vi "Test StateMachine API.vi"() -> ()   [LabVIEW 2020]
doc: "StateMachine API Tester.\n\n<b>Note:</b> This VI was modified by the <b>Validate DQMH Module</b> tool to add the 'Show Main VI Diagram on Init' functionality included in DQMH 6.1.\n\n<b>Note:</b> This VI was modified by the <b>Validate DQMH Module</b> tool to upgrade its Error Reported event frame to use an improved mechanism for displaying error information.\n\n____\nHAMPEL SOFTWARE ENGINEERING v2.6.0 (2023-12-19 10:54)"
uses:
  Libraries/hse-libraries/Source/hse-dqmh/Controls/Module Display Scenarios.ctl
  HSE-SM/SM_Transitions.ctl
  <vilib>/Utility/error.llb/DialogType.ctl
  <vilib>/Hampel Software Engineering/HSE Logger/LogRecord/LogRecord.lvclass/LogRecord.ctl
  StateMachine.lvlib
  Libraries/hse-libraries/Source/hse-dqmh/hse-dqmh.lvlib
  <vilib>/Hampel Software Engineering/HSE Logger/LogRecord/LogRecord.lvclass
  <vilib>/Hampel Software Engineering/HSE Logger/hse-logger.lvlib
  HSE-SM/HSE-State-Machine.lvlib
panel:
  in  "Show Main VI Diagram on Init (F)":bool
  in  "DEMO Transition to inject":T1
  in  "DEMO Inject Transition":bool
  in  "Scenario":T2
  in  "Request UI Display":bool
  in  "Prepare":bool
  in  "Configure":bool
  in  "Show Block Diagram":bool
  in  "Stop Module":bool
  in  "Start Module":bool
  in  "Hide Module Panel":bool
  in  "Show Module Panel":bool
  out "Status":string
  out "Module Running?":bool
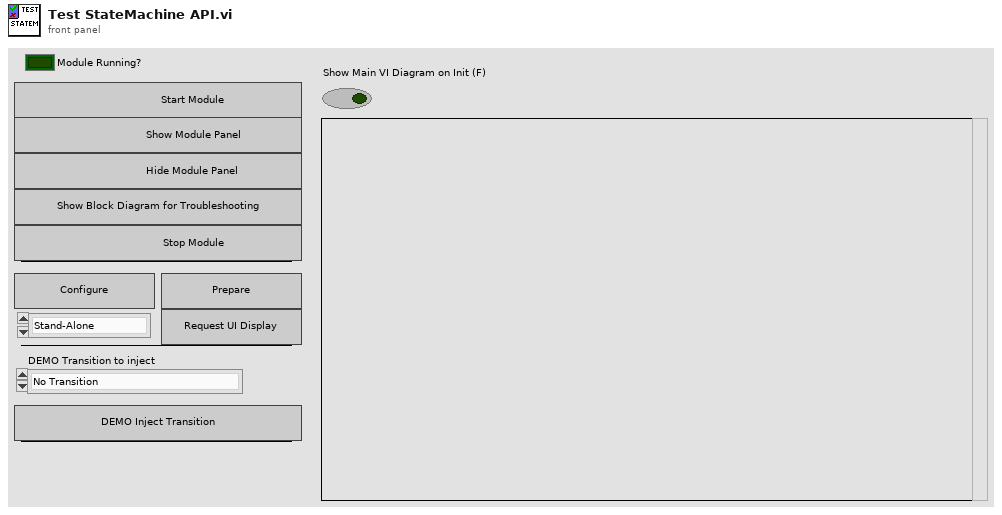
[diagram p1: front panel]
types:
  T1 = typedef "StateMachine.lvlib/HSE-State-Machine.lvlib/SM_Transitions.ctl" = enum16{"No Transition", "Exception", "Reset", "Initialization finished", "Process started", "Trigger detected", "Exit"}
  T2 = typedef "hse-dqmh.lvlib/Module Display Scenarios.ctl" = enum16{"Stand-Alone", "Managed"}
  T3 = typedef "StateMachine.lvlib/Broadcast Events--cluster.ctl" = cluster{"Module Did Init":refnum<user-event>, "Status Updated":refnum<user-event>, "Error Reported":refnum<user-event>, "Module Did Stop":refnum<user-event>, "Update Module Execution Status":refnum<user-event>, "System Message":refnum<user-event>, "DEMO Updated UI State":refnum<user-event>}
  T4 = typedef "DialogType.ctl" = u16
  T5 = typedef "hse-dqmh.lvlib/System Message Source.ctl" = enum16{"module", "application", "network"}
  T6 = typedef "hse-logger.lvlib/LogLevel.ctl" = enum16{"DEBUG", "INFO", "WARNING", "ERROR", "CRITICAL"}
  T7 = typedef "StateMachine.lvlib/HSE-State-Machine.lvlib/SM_States.ctl" = enum16{"No State - Error", "Error - Waiting For Action", "Initialising", "Standing by (idle)", "Waiting for External Trigger", "Polling for Signal Change", "Exiting"}
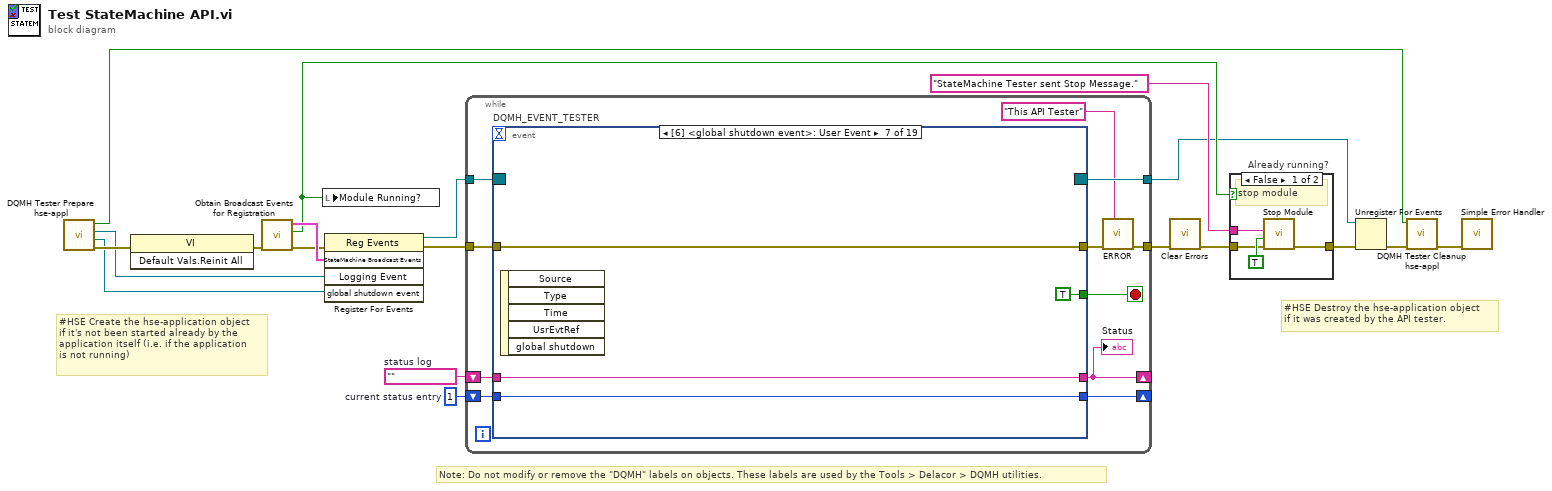
[diagram p0: block diagram]
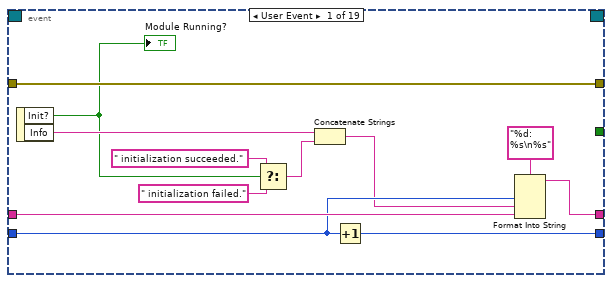
[diagram p3: hidden frame]
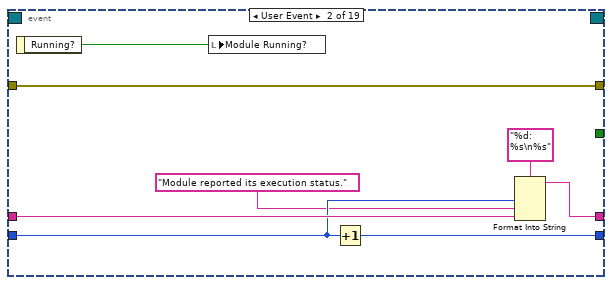
[diagram p4: hidden frame]
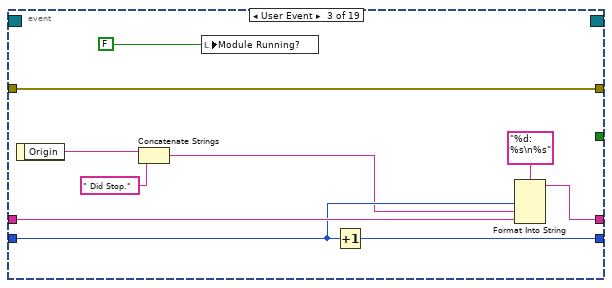
[diagram p5: hidden frame]
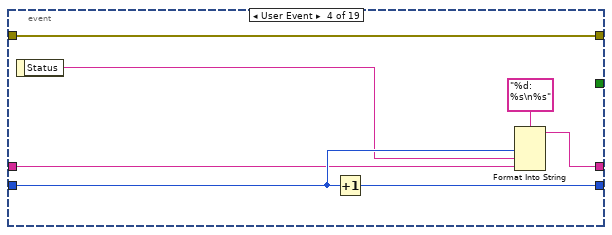
[diagram p6: hidden frame]
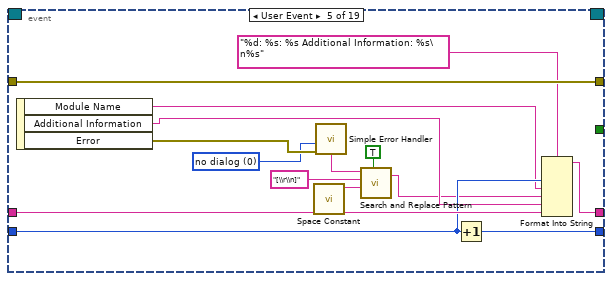
[diagram p7: hidden frame]
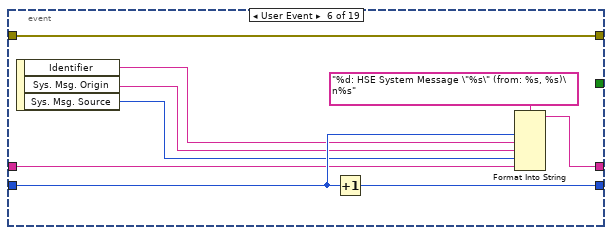
[diagram p8: hidden frame]
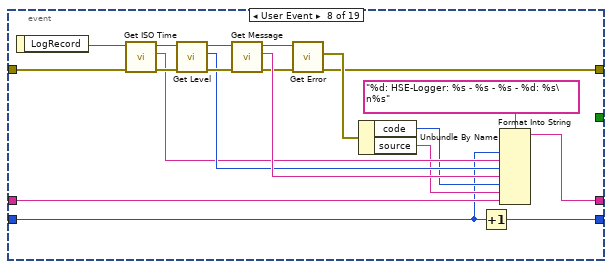
[diagram p9: hidden frame]
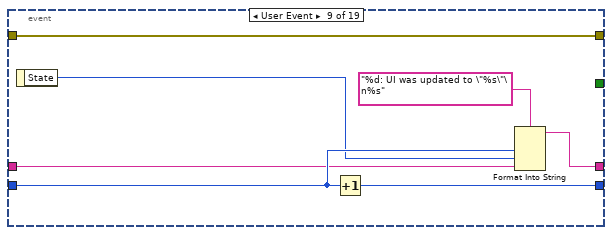
[diagram p10: hidden frame]
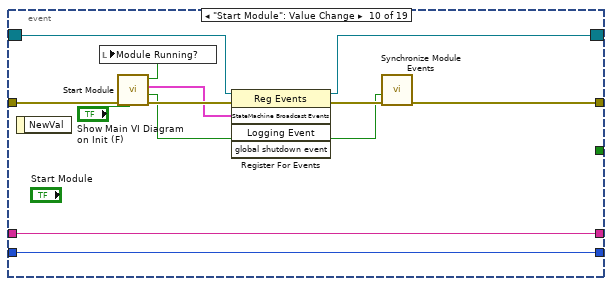
[diagram p11: hidden frame]
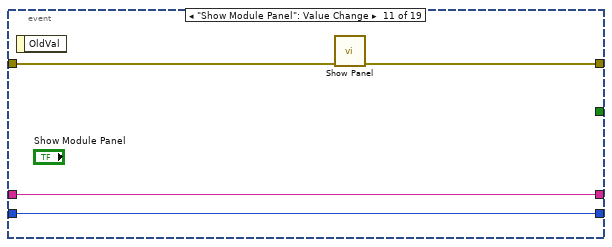
[diagram p12: hidden frame]
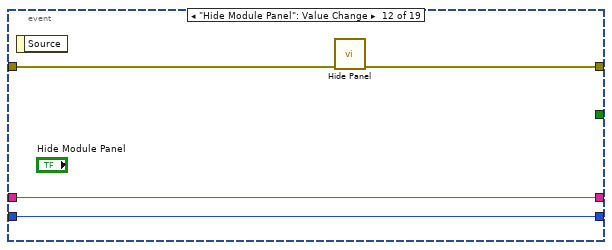
[diagram p13: hidden frame]
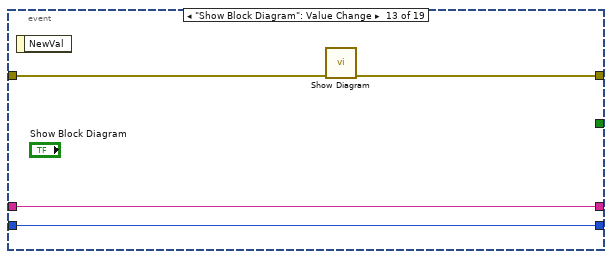
[diagram p14: hidden frame]
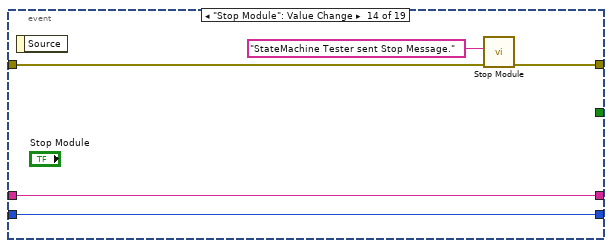
[diagram p15: hidden frame]
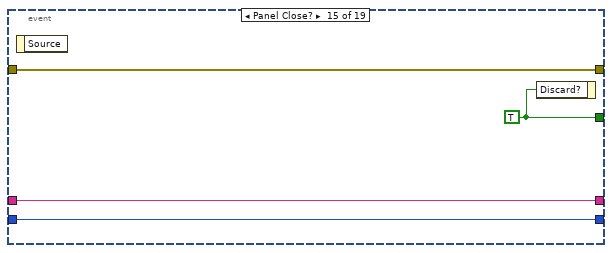
[diagram p16: hidden frame]
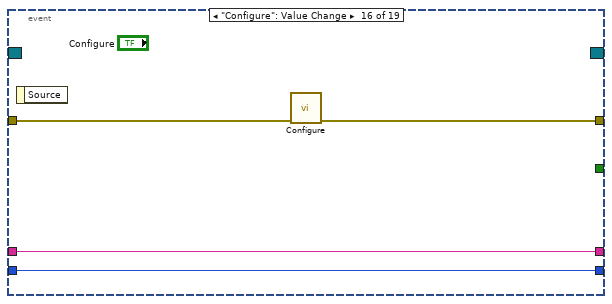
[diagram p17: hidden frame]
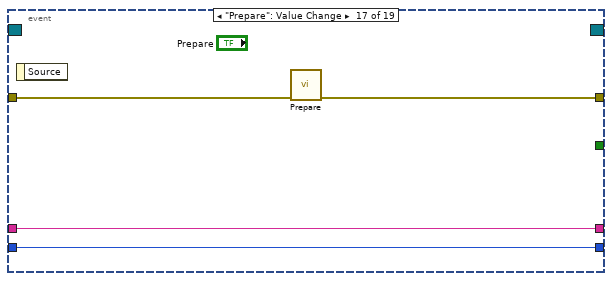
[diagram p18: hidden frame]
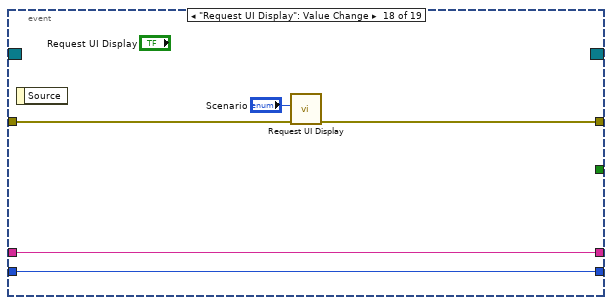
[diagram p19: hidden frame]
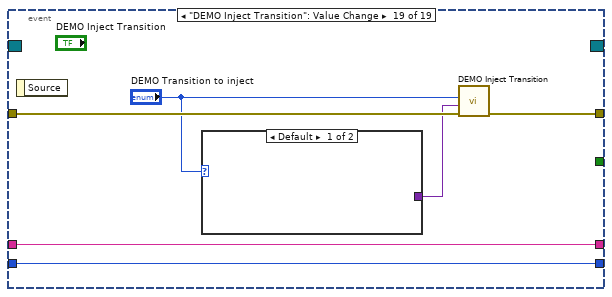
[diagram p20: hidden frame]
diagram:
  w15 = 1  # current status entry
  w16 = ""  # status log
  # "#HSE Destroy the hse-application object\nif it was created by the API tester."
  # "#HSE Create the hse-application object\nif it's not been started already by the \napplication itself (i.e. if the application\nis not running)"
  # "Note: Do not modify or remove the \"DQMH\" labels on objects. These labels are used by the Tools > Delacor > DQMH utilities."
  n1 = call "DQMH Tester Prepare hse-appl.vi"() -> ("error out"=w6:errorcluster, "global shutdown event"=w1:refnum<user-event>, "Logging Event"=w5:refnum<user-event>, "Started?"=w4:bool)  [unwired: 8 in]
  n2 = invoke class="VI" method="Default Vals.Reinit All"(error in=w6) -> (error out=w9:errorcluster)  [unwired: 2 in, 2 out]
  n3 = call "Obtain Broadcast Events for Registration.vi"("error in (no error)"=w9) -> ("error out"=w8:errorcluster, "Already running?"=w7:bool, "StateMachine Broadcast Events"=w13:T3)  [unwired: 8 in]
  n4 = local write "Module Running?"(w7) -> ()
  n5 = register-events(error in=w8, w13, w5, w1) -> (reference out=w12:refnum<event-registration>, error out=w14:errorcluster)  [unwired: 1 in]
  n6 = while {
    tunnel: w12 -> [w30]
    tunnel: [w21] -> w10
    shift-right: [w26] -> _
    shift-left: w16 -> [w28]
    shift-right: [w27] -> _
    shift-left: w15 -> [w29]
    tunnel: w14 -> [w25]
    tunnel: [w24] -> w2
    stop <- w23 stop-if-true
    n7 = event "DQMH_EVENT_TESTER" shown="[6] <global shutdown event>: User Event" {
      selector: w30 -> [_ _ _ _ _ _ _ _ _ w127 _ _ _ _ _ _ _ _ _]
      dyn-events: [_ _ _ _ _ _ _ _ _ w126 _ _ _ _ _ _ _ _ _] -> w24
      timeout: _ -> [_ _ _ _ _ _ _ _ _ _ _ _ _ _ _ _ _ _ _]
      tunnel: [_ _ _ _ _ _ TRUE ("Discard?") _ _ _ _ _ _ _ w154 _ _ _ _] -> w23
      tunnel: [w42 w44 w51 w61 w82 w86 w95 w96 w121 w125 w137 w141 w142 w148 w151 w155 w159 w164 w170] -> w22
      tunnel: w29 -> [w39 w48 w58 w64 w79 w88 w93 w99 w120 w130 w135 w139 w143 w149 w152 w156 w160 w165 w171]
      tunnel: w28 -> [w40 w49 w59 w63 w81 w85 w94 w100 w118 w131 w136 w140 w144 w150 w153 w157 w161 w166 w172]
      tunnel: [w37 w46 w56 w65 w80 w89 w94 w97 w117 w131 w136 w140 w144 w150 w153 w157 w161 w166 w172] -> w26
      tunnel: [w38 w47 w57 w67 w78 w91 w93 w98 w120 w130 w135 w139 w143 w149 w152 w156 w160 w165 w171] -> w27
      tunnel: w25 -> [w42 w44 w51 w61 w82 w86 w95 w102 w121 w124 w134 w138 w145 w146 w151 w158 w162 w167 w173]
      event User Event {
        n8 = event-data() -> ("Init?"=w34:bool, "Info"=w36:string)  [unwired: 1 in]
        "Module Running?" <- w34
        n9 = Select(t=" initialization succeeded.", s=w34, f=" initialization failed.") -> (s? t:f=w31:string)
        n10 = Concatenate Strings(w36, w31) -> (w35:string)
        n11 = Increment(x=w39) -> (x+1=w38:i32)
        n12 = Format Into String(format string="%d: %s\n%s", w39, w35, w40) -> (resulting string=w37:string)  [unwired: 2 in, 1 out]
      }
      event User Event {
        n13 = event-data() -> ("Running?"=w43:bool)  [unwired: 1 in]
        n14 = local write "Module Running?"(w43) -> ()
        n15 = Increment(x=w48) -> (x+1=w47:i32)
        n16 = Format Into String(format string="%d: %s\n%s", w48, "Module reported its execution status.", w49) -> (resulting string=w46:string)  [unwired: 2 in, 1 out]
      }
      event User Event {
        n17 = event-data() -> ("Origin"=w55:string)  [unwired: 1 in]
        n18 = Concatenate Strings(w55, " Did Stop.") -> (w54:string)
        n19 = local write "Module Running?"(FALSE ("Module Did Init?")) -> ()
        n20 = Increment(x=w58) -> (x+1=w57:i32)
        n21 = Format Into String(format string="%d: %s\n%s", w58, w54, w59) -> (resulting string=w56:string)  [unwired: 2 in, 1 out]
      }
      event User Event {
        n22 = event-data() -> ("Status"=w62:string)  [unwired: 1 in]
        n23 = Increment(x=w64) -> (x+1=w67:i32)
        n24 = Format Into String(format string="%d: %s\n%s", w64, w62, w63) -> (resulting string=w65:string)  [unwired: 2 in, 1 out]
      }
      event User Event {
        w74 = T4 0 items=["no dialog", "OK message", "continue or stop message", "OK message + warnings", "continue/stop + warnings"] ("type of dialog (OK msg:1)")
        n25 = event-data() -> ("Module Name"=w75:string, "Additional Information"=w76:string, "Error"=w77:errorcluster)  [unwired: 1 in]
        n26 = call <vilib>:"Space Constant.vi"() -> ("String"=w70:string)
        n27 = call <vilib>:"Simple Error Handler.vi"("type of dialog (OK msg:1)"=w74, "error in (no error)"=w77) -> ("message"=w73:string)  [unwired: 3 in, 4 out]
        n28 = call <vilib>:"Search and Replace Pattern.vi"("string"=w73, "regular expression (\"\")"="[\\r\\n]" ("regular expression (\"\")"), "replace string (\"\")"=w70, "replace all? (F)"=TRUE ("replace all CR/LF with spaces")) -> ("result string"=w72:string)  [unwired: 1 in, 1 out]
        n29 = Increment(x=w79) -> (x+1=w78:i32)
        n30 = Format Into String(format string="%d: %s: %s Additional Information: %s\n%s", w79, w75, w72, w76, w81) -> (resulting string=w80:string)  [unwired: 2 in, 1 out]
      }
      event User Event {
        n31 = event-data() -> ("Identifier"=w87:string, "Sys. Msg. Origin"=w83:string, "Sys. Msg. Source"=w84:T5)  [unwired: 1 in]
        n32 = Increment(x=w88) -> (x+1=w91:i32)
        n33 = Format Into String(format string="%d: HSE System Message \"%s\" (from: %s, %s)\n%s", w88, w87, w83, w84, w85) -> (resulting string=w89:string)  [unwired: 2 in, 1 out]
      }
      event User Event {
        n34 = event-data() -> ()  [unwired: 1 in, 5 out]
      }
      event User Event {
        n35 = event-data() -> ("LogRecord"=w101:refnum<class "LogRecord.lvclass">)  [unwired: 1 in]
        n36 = call <vilib>:"Get ISO Time.vi"("error in"=w102, "LogRecord in"=w101) -> ("error out"=w107:errorcluster, "ISO Time"=w106:string, "LogRecord out"=w109:refnum<class "LogRecord.lvclass">)  [unwired: 7 in]
        n37 = call <vilib>:"Get Level.vi"("error in"=w107, "LogRecord in"=w109) -> ("error out"=w110:errorcluster, "Level"=w108:T6, "LogRecord out"=w111:refnum<class "LogRecord.lvclass">)  [unwired: 7 in]
        n38 = call <vilib>:"Get Message.vi"("error in"=w110, "LogRecord in"=w111) -> ("error out"=w112:errorcluster, "Message"=w115:string, "LogRecord out"=w113:refnum<class "LogRecord.lvclass">)  [unwired: 7 in]
        n39 = call <vilib>:"Get Error.vi"("error in"=w112, "LogRecord in"=w113) -> ("error out"=w96:errorcluster, "Error"=w114:errorcluster)  [unwired: 7 in, 1 out]
        n40 = Unbundle By Name(w114) -> ("code"=w104:i32, "source"=w105:string)
        n41 = Increment(x=w99) -> (x+1=w98:i32)
        n42 = Format Into String(format string="%d: HSE-Logger: %s - %s - %s - %d: %s\n%s", w99, w106, w108, w115, w104, w105, w100) -> (resulting string=w97:string)  [unwired: 2 in, 1 out]
      }
      event User Event {
        n43 = event-data() -> ("State"=w119:T7)  [unwired: 1 in]
        n44 = Increment(x=w120) -> ()  [unwired: 1 out]
        n45 = Format Into String(format string="%d: UI was updated to \"%s\"\n%s", w120, w119, w118) -> (resulting string=w117:string)  [unwired: 2 in, 1 out]
      }
      event "Start Module": Value Change {
        n46 = event-data() -> ()  [unwired: 1 in, 1 out]
        n47 = call "Start Module.vi"("Show Main VI Diagram on Init (F)"="Show Main VI Diagram on Init (F)", "error in (no error)"=w124) -> ("error out"=w132:errorcluster, "Wait for Event Sync?"=w129:bool, "StateMachine Broadcast Events"=w128:T3, "Module Was Already Running?"=w123:bool)  [unwired: 6 in]
        n48 = local write "Module Running?"(w123) -> ()
        n49 = register-events(reference=w127, error in=w132, w128) -> (reference out=w126:refnum<event-registration>, error out=w133:errorcluster)  [unwired: 2 in]
        n50 = call "Synchronize Module Events.vi"("error in (no error)"=w133, "Wait for Event Sync?"=w129) -> ("error out"=w125:errorcluster)  [unwired: 9 in]
      }
      event "Show Module Panel": Value Change {
        n51 = event-data() -> ()  [unwired: 1 in, 1 out]
        n52 = call "Show Panel.vi"("error in (no error)"=w134) -> ("error out"=w137:errorcluster)  [unwired: 10 in]
      }
      event "Hide Module Panel": Value Change {
        n53 = event-data() -> ()  [unwired: 1 in, 1 out]
        n54 = call "Hide Panel.vi"("error in (no error)"=w138) -> ("error out"=w141:errorcluster)  [unwired: 10 in]
      }
      event "Show Block Diagram": Value Change {
        n55 = event-data() -> ()  [unwired: 1 in, 1 out]
        n56 = call "Show Diagram.vi"("error in (no error)"=w145) -> ("error out"=w142:errorcluster)  [unwired: 10 in]
      }
      event "Stop Module": Value Change {
        n57 = event-data() -> ()  [unwired: 1 in, 1 out]
        n58 = call "Stop Module.vi"("error in (no error)"=w146, "Origin"="StateMachine Tester sent Stop Message.") -> ("error out"=w148:errorcluster)  [unwired: 9 in]
      }
      event Panel Close? {
        w154 = TRUE ("Discard?")
        n59 = event-data() -> ()  [unwired: 1 in, 1 out]
        n60 = event-data("Discard?"=w154) -> ()  [unwired: 1 in, 1 out]
      }
      event "Configure": Value Change {
        n61 = event-data() -> ()  [unwired: 1 in, 1 out]
        n62 = call "Configure.vi"("error in (no error)"=w158) -> ("error out"=w155:errorcluster)  [unwired: 10 in]
      }
      event "Prepare": Value Change {
        n63 = event-data() -> ()  [unwired: 1 in, 1 out]
        n64 = call "Prepare.vi"("error in (no error)"=w162) -> ("error out"=w159:errorcluster)  [unwired: 10 in]
      }
      event "Request UI Display": Value Change {
        n65 = event-data() -> ()  [unwired: 1 in, 1 out]
        n66 = call "Request UI Display.vi"("error in (no error)"=w167, "Scenario"="Scenario") -> ("error out"=w164:errorcluster)  [unwired: 8 in, 1 out]
      }
      event "DEMO Inject Transition": Value Change {
        n67 = event-data() -> ()  [unwired: 1 in, 1 out]
        n68 = case shown="Default" "DEMO Transition to inject" {
          tunnel: [_ w174] -> w169
          frame Default {
          }
          frame "Exception" {
            n69 = To Variant(anything=errorcluster {"status"=TRUE, "code"=500001, "source"="DEMO simulated error"} ("error out")) -> (Variant=w174:variant)
          }
        }
        n70 = call "DEMO Inject Transition.vi"("error in (no error)"=w173, "Data"=w169, "Transition"="DEMO Transition to inject") -> ("error out"=w170:errorcluster)  [unwired: 8 in]
      }
    }
    "Status" <- w26
    n71 = call <vilib>:"ERROR.vi"("Message"="This API Tester" ("Origin"), "error in"=w22) -> ("error out"=w21:errorcluster)  [unwired: 9 in]
  }
  n72 = call <vilib>:"Clear Errors.vi"("error in (no error)"=w10) -> ("error out"=w11:errorcluster)  [unwired: 5 in, 1 out]
  n73 = case "Already running?" shown="False" w7 {
    tunnel: [w179 w180] -> w18
    tunnel: "StateMachine Tester sent Stop Message." ("Origin") -> [w178 _]
    tunnel: w11 -> [w176 w180]
    frame False {
      # "stop module"
      n74 = call "Stop Module.vi"("error in (no error)"=w176, "Wait for Module to Stop? (F)"=TRUE ("Wait for Module to stop?"), "Origin"=w178) -> ("error out"=w179:errorcluster)  [unwired: 8 in]
    }
    frame True {
      # "don't stop"
    }
  }
  n75 = Unregister For Events(event registration refnum=w2, error in=w18) -> (error out=w19:errorcluster)
  n76 = call "DQMH Tester Cleanup hse-appl.vi"("error in"=w19, "Stop?"=w4) -> ("error out"=w3:errorcluster)  [unwired: 9 in]
  n77 = call <vilib>:"Simple Error Handler.vi"("error in (no error)"=w3) -> ()  [unwired: 4 in, 5 out]
